vi "Redo.vi"(8 "error in (no error)":errorcluster, 11 "UndoObject in":refnum<class "UndoObject.lvclass">) -> (0 "error out":errorcluster, 2 "Ctrl Val.Get All":T1[](array[typedef]), 3 "UndoObject out":refnum<class "UndoObject.lvclass">, 4 "Redo Enable":bool, 6 "Undo Enable":bool)   [LabVIEW 2015, in "UndoLibrary.lvlib" / "UndoObject.lvclass"]
doc: "This VI stores the values to perform the redo action."
uses:
  UndoObject.lvclass
  Support VIs/DataClass/Controls/cluster_Control Value.ctl
  UndoObject.lvclass/UndoObject.ctl
  Support VIs/DataClass/DataObject.lvclass/DataObject.ctl
  Support VIs/DataClass/DataObject.lvclass
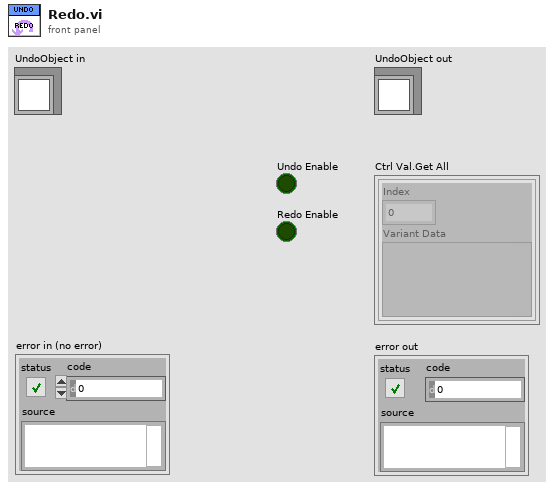
[diagram p1: front panel]
types:
  T1 = typedef "UndoLibrary.lvlib/DataObject.lvclass/cluster_Control Value.ctl" = cluster{"Index":i32, "Variant Data":variant}
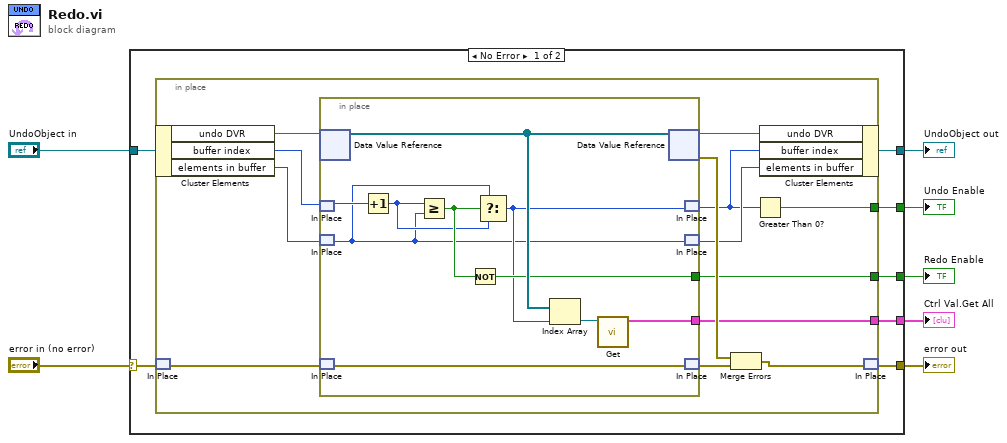
[diagram p0: block diagram]
diagram:
  n1 = case shown="No Error" "error in (no error)" {
    selector: "error in (no error)" -> [w13 w39]
    tunnel: [w12 w39] -> w7
    tunnel: "UndoObject in" -> [w11 w38]
    tunnel: [w14 _] -> w5
    tunnel: [w10 w38] -> w1
    tunnel: [w9 _] -> w4
    tunnel: [w8 _] -> w3
    frame No Error {
      n2 = in-place {
        in-place-border: [w18] -> w14
        in-place-border: [w15] -> w9
        in-place-border: [w17] -> w8
        n3 = in-place-cluster #1(w11) -> ("undo DVR"=w25:refnum<data-value>, "buffer index"=w21:i32, "elements in buffer"=w20:i32)
        n4 = in-place-match #2(w13) -> (w27:errorcluster)
        n5 = in-place {
          in-place-border: [w34] -> w17
          in-place-border: [w28] -> w18
          n6 = in-place-dvr #3(w25) -> (w35:refnum<class "DataObject.lvclass">[])  [unwired: 1 out]
          n7 = in-place-match #4(w21) -> (w33:i32)
          n8 = in-place-match #5(w20) -> (w31:i32)
          n9 = in-place-match #6(w27) -> (w30:errorcluster)
          n10 = Increment(x=w33) -> (x+1=w36:i32)
          n11 = Greater Or Equal?(x=w36, y=w31) -> (x >= y?=w37:bool)
          n12 = Not(x=w37) -> (.not. x?=w34:bool)
          n13 = Select(t=w31, s=w37, f=w36) -> (s? t:f=w32:i32)
          n14 = Index Array(array=w35, index=w32) -> (element=w29:refnum<class "DataObject.lvclass">)
          n15 = call "Get.vi"("DataObject in"=w29) -> ("Conrol Value[]"=w28:T1[])  [unwired: 9 in, 1 out]
          n16 = in-place-dvr #3(w35) -> (w24:refnum<data-value>, w22:errorcluster)
          n17 = in-place-match #4(w32) -> (w16:i32)
          n18 = in-place-match #5(w31) -> (w19:i32)
          n19 = in-place-match #6(w30) -> (w26:errorcluster)
        }
        n20 = Merge Errors(w22, w26) -> (w23:errorcluster)
        n21 = Greater Than 0?(x=w16) -> (x > 0?=w15:bool)
        n22 = in-place-cluster #1("undo DVR"=w24, "buffer index"=w16, "elements in buffer"=w19) -> (w10:refnum<class "UndoObject.lvclass">)
        n23 = in-place-match #2(w23) -> (w12:errorcluster)
      }
    }
    frame Error {
    }
  }
  "error out" <- w7
  "Ctrl Val.Get All" <- w5
  "Undo Enable" <- w4
  "Redo Enable" <- w3
  "UndoObject out" <- w1
